vi "SerializeNode.vi"(8 "error in (no error)":errorcluster, 11 "Node in":refnum<class "DirectoryMetadata.lvclass">) -> (0 "error out":errorcluster, 2 "Serialized String":string, 3 "Node out":refnum<class "DirectoryMetadata.lvclass">)   [LabVIEW 2017, in "DirectoryMetadata.lvclass"]
uses:
  DirectoryMetadata.lvclass
  DirectoryMetadata.lvclass/DirectoryMetadata.ctl
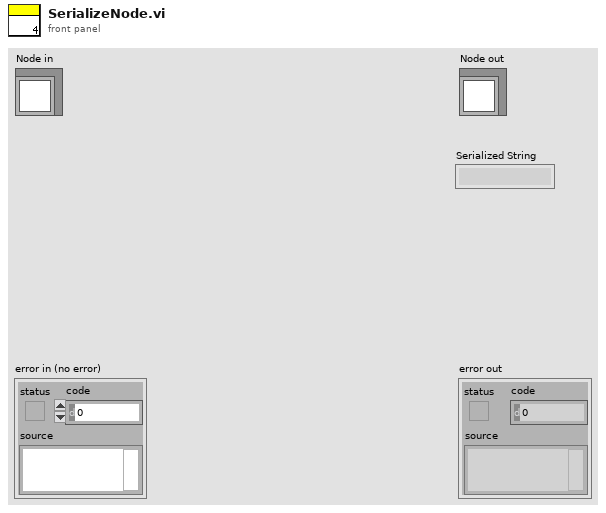
[diagram p1: front panel]
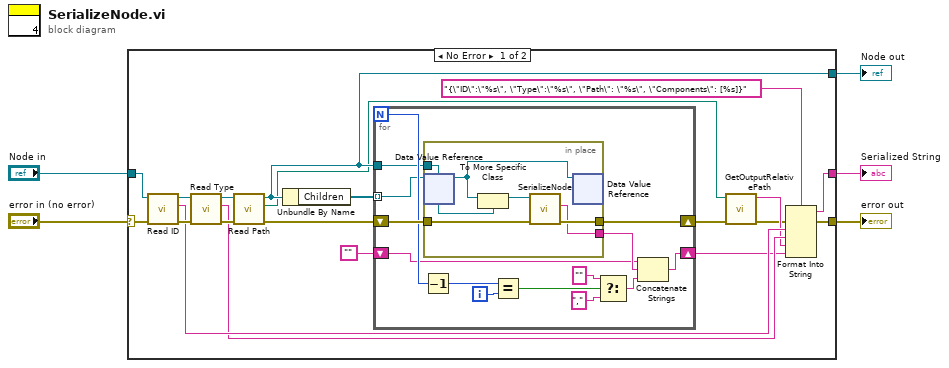
[diagram p0: block diagram]
diagram:
  n1 = case shown="No Error" "error in (no error)" {
    selector: "error in (no error)" -> [w22 w47]
    tunnel: [w8 w47] -> w4
    tunnel: [w13 w46] -> w2
    tunnel: "Node in" -> [w20 w46]
    tunnel: [w15 _] -> w1
    frame No Error {
      n2 = call "Read ID.vi"("error in (no error)"=w22, "ClassMetadata in"=w20) -> ("error out"=w25:errorcluster, "ID"=w18:string, "ClassMetadata out"=w24:refnum<class "DirectoryMetadata.lvclass">)  [unwired: 7 in]
      n3 = call "Read Type.vi"("error in (no error)"=w25, "ClassMetadata in"=w24) -> ("error out"=w23:errorcluster, "Type"=w17:string, "ClassMetadata out"=w21:refnum<class "DirectoryMetadata.lvclass">)  [unwired: 7 in]
      n4 = call "Read Path.vi"("error in (no error)"=w23, "ClassMetadata in"=w21) -> ("error out"=w14:errorcluster, "Path"=w11:path, "ClassMetadata out"=w13:refnum<class "DirectoryMetadata.lvclass">)  [unwired: 7 in]
      n5 = Unbundle By Name(w13) -> ("Children"=w12:refnum<data-value>[])
      n6 = for {
        N -> [w37]
        tunnel: w12 -> [w27] mode=indexing
        shift-right: [w36] -> w9
        shift-left: w14 -> [w39]
        shift-right: [w29] -> w16
        shift-left: "" -> [w28]
        tunnel: w13 -> [w26]
        i -> [w38]
        n7 = Decrement(x=w37) -> (x-1=w35:i32)
        n8 = in-place {
          in-place-border: w39 -> [w45]
          in-place-border: [w44] -> w36
          in-place-border: [w43] -> w31
          in-place-border: w26 -> [w42]
          n9 = in-place-dvr #1(w27) -> (w40:refnum<class>)  [unwired: 1 out]
          n10 = To More Specific Class(target class=w42, reference=w40) -> (specific class reference=w41:refnum<class "DirectoryMetadata.lvclass">)  [unwired: 1 in, 1 out]
          n11 = call "SerializeNode.vi"("error in (no error)"=w45, "Node in"=w41) -> ("error out"=w44:errorcluster, "Serialized String"=w43:string)  [unwired: 7 in, 1 out]
          n12 = in-place-dvr #1(w40) -> ()  [unwired: 2 out]
        }
        n13 = Equal?(x=w35, y=w38) -> (x = y?=w34:bool)
        n14 = Select(t="" ("string"), s=w34, f="," ("string")) -> (s? t:f=w30:string)
        n15 = Concatenate Strings(w28, w31, w30) -> (w29:string)
      }
      n16 = call "GetOutputRelativePath.vi"("error in (no error)"=w9, "Path"=w11) -> ("error out"=w7:errorcluster, "Output relative path"=w10:string)  [unwired: 8 in]
      n17 = Format Into String(format string="{\"ID\":\"%s\", \"Type\":\"%s\", \"Path\": \"%s\", \"Components\": [%s]}", error in=w7, w18, w17, w10, w16) -> (resulting string=w15:string, error out=w8:errorcluster)  [unwired: 1 in]
    }
    frame Error {
    }
  }
  "error out" <- w4
  "Node out" <- w2
  "Serialized String" <- w1
